vi "PH_IEEE1394Camera.set Cam Attributes to GUI.vi"(0 "VI in":refnum<vi>, 5 "error in (no error)":errorcluster) -> (14 "VI out":refnum<vi>, 19 "error out":errorcluster)   [LabVIEW 2014, in "PH_IEEE1394Camera.lvlib"]
uses:
  PH_IEEE1394Camera.lvlib
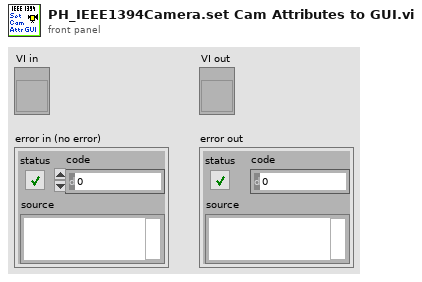
[diagram p1: front panel]
types:
  T1 = typedef "PH_IEEE1394Camera.lvlib/PH_IEEE1394Camera.i attribute.ctl" = cluster{"Gui Refs":cluster{"Brightness":refnum<vi>, "Shutter":refnum<vi>, "Gain":refnum<vi>, "Center of Gravity":refnum<vi>, "Supported Video Modes":refnum<vi>, "Trigger Polarity":refnum<vi>, "Trigger Mode":refnum<vi>, "Trigger Timeout":refnum<vi>, "Bit Depth":refnum<vi>, "Video Mode":refnum<vi>, "Top":refnum<vi>, "Bottom":refnum<vi>, "Left":refnum<vi>, "Right":refnum<vi>, "Set ROI to Maximum":refnum<vi>, "Camera Details":refnum<vi>, "Current Cam Attributes":refnum<vi>, "Attribute to set":refnum<vi>, "Num Value":refnum<vi>, "String Value":refnum<vi>, "Bool Value":refnum<vi>, "Set Cam Attribute":refnum<vi>}, "Cam":cluster{"IMAQ1394 Session":T2, "Camera Details":T3}, "Current Attributes":T4[], "Supported Video Modes ":cluster{"Video Mode":u32, "Video Mode Name":string}[], "Wanted Attributes":cluster{"Name":string, "Num Value":dbl, "String Value":string, "Boolean Value":bool}[], "Cam Attributes":T6}
  T2 = typedef "IMAQdx.ctl" = refnum<k21>
  T3 = typedef "PH_IEEE1394Camera.lvlib/PH_IEEE1394Camera.Cam Details.ctl" = cluster{"Model":string, "Serial Number":dbl, "Cam name (Machinery)":string, "Bus Type":string}
  T4 = typedef "PH_IEEE1394Camera.lvlib/PH_IEEE1394Camera.Cam Attribute.ctl" = cluster{"Information":cluster{"Type":T5, "Readable":bool, "Writable":bool, "Name":string}, "Num Value":dbl, "String Value":string, "Maximum":dbl, "Minimum":dbl, "Units":string, "Description":string, "EnumStrings[]":string[], "EnumValues[]":u32[], "Boolean Value":bool}
  T5 = typedef "NI_Vision_Acquisition_Software.lvlib/IMAQdx Attribute Type.ctl" = enum32{"U32", "I64", "DBL", "String", "Enum", "Bool", "Command"}
  T6 = typedef "PH_IEEE1394Camera.lvlib/PH_IEEE1394Camera.Relevant Cam Attributes.ctl" = cluster{"Video Mode":cluster{"Name":string, "Index":i32}, "Brightness":cluster{"Name":string, "Index":i32}, "Gain":cluster{"Name":string, "Index":i32}, "Shutter":cluster{"Name":string, "Index":i32}, "Trigger Pol":cluster{"Name":string, "Index":i32}, "Trigger Mode":cluster{"Name":string, "Index":i32}, "Timeout":cluster{"Name":string, "Index":i32}, "Bit Depth":cluster{"Name":string, "Index":i32}, "Pixel Bits":cluster{"Name":string, "Index":i32}, "Pixel Bytes":cluster{"Name":string, "Index":i32}, "Left":cluster{"Name":string, "Index":i32}, "Right":cluster{"Name":string, "Index":i32}, "Top":cluster{"Name":string, "Index":i32}, "Bottom":cluster{"Name":string, "Index":i32}}
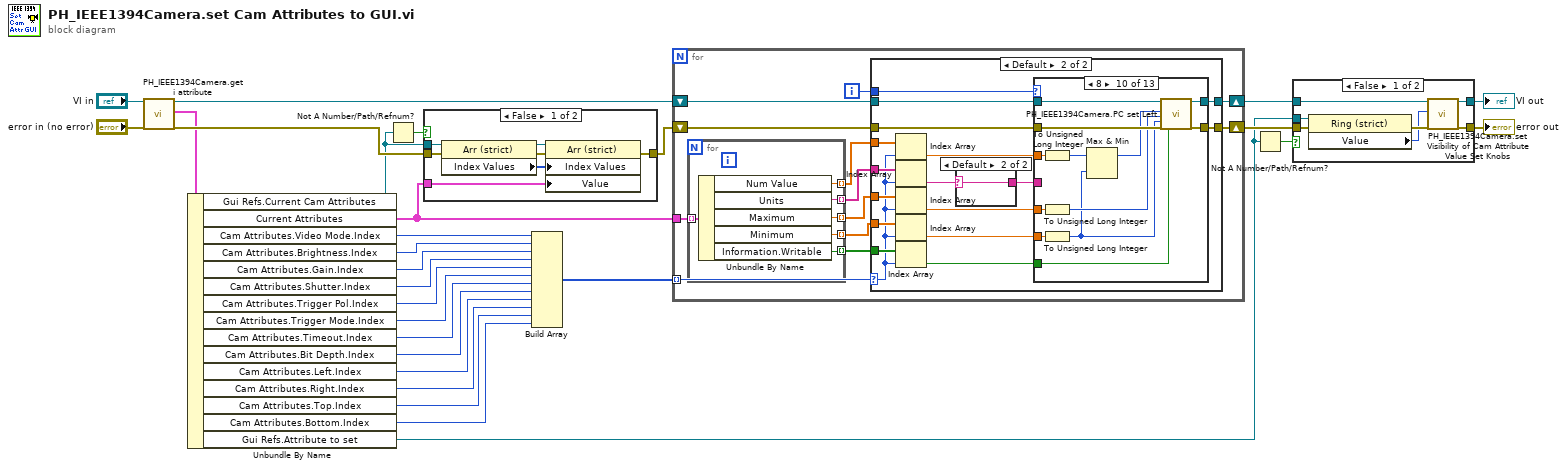
[diagram p0: block diagram]
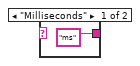
[diagram p4: hidden frame]
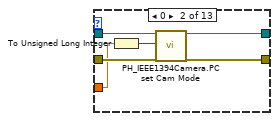
[diagram p6: hidden frame]
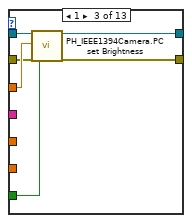
[diagram p7: hidden frame]
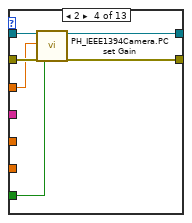
[diagram p8: hidden frame]
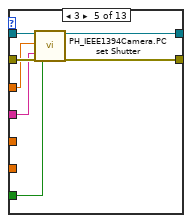
[diagram p9: hidden frame]
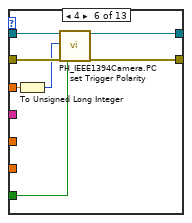
[diagram p10: hidden frame]
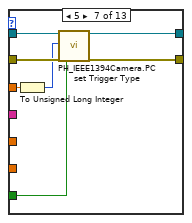
[diagram p11: hidden frame]
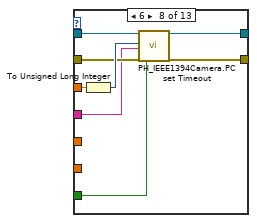
[diagram p12: hidden frame]
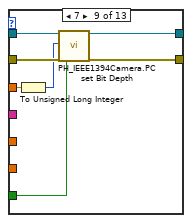
[diagram p13: hidden frame]
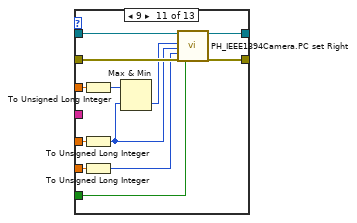
[diagram p14: hidden frame]
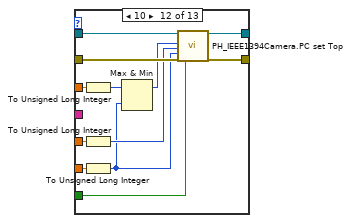
[diagram p15: hidden frame]
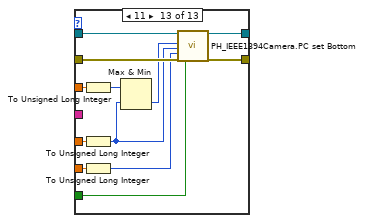
[diagram p16: hidden frame]
diagram:
  n1 = call "PH_IEEE1394Camera.get i attribute.vi"("i ref in"="VI in", "error in (no error)"="error in (no error)") -> ("i ref out"=w11:refnum<vi>, "i attribute"=w1:T1, "error out"=w14:errorcluster)  [unwired: 15 in]
  n2 = Unbundle By Name(w1) -> ("Gui Refs.Current Cam Attributes"=w13:refnum<vi>, "Current Attributes"=w9:T4[], "Cam Attributes.Video Mode.Index"=w26:i32, "Cam Attributes.Brightness.Index"=w25:i32, "Cam Attributes.Gain.Index"=w24:i32, "Cam Attributes.Shutter.Index"=w23:i32, "Cam Attributes.Trigger Pol.Index"=w22:i32, "Cam Attributes.Trigger Mode.Index"=w21:i32, "Cam Attributes.Timeout.Index"=w20:i32, "Cam Attributes.Bit Depth.Index"=w19:i32, "Cam Attributes.Left.Index"=w18:i32, "Cam Attributes.Right.Index"=w17:i32, "Cam Attributes.Top.Index"=w16:i32, "Cam Attributes.Bottom.Index"=w15:i32, "Gui Refs.Attribute to set"=w2:refnum<vi>)
  n3 = Not A Number/Path/Refnum?(number/path/refnum=w13) -> (NaN/Path/Refnum?=w12:bool)
  n4 = case shown="False" w12 {
    tunnel: [w32 w36] -> w10
    tunnel: w9 -> [w29 _]
    tunnel: w14 -> [w35 w36]
    tunnel: w13 -> [w34 _]
    frame False {
      n5 = property class="Arr (strict)"(reference=w34, error in=w35) -> (reference out=w30:refnum<vi>, error out=w33:errorcluster, "Index Values"=w31:u32[])
      n6 = property class="Arr (strict)"(reference=w30, error in=w33, "Index Values"=w31, "Value"=w29) -> (error out=w32:errorcluster)  [unwired: 1 out]
    }
    frame True {
    }
  }
  n7 = Build Array(w26, w25, w24, w23, w22, w21, w20, w19, w18, w17, w16, w15) -> (w8:i32[])
  n8 = for {
    shift-right: [w47] -> w7
    shift-left: w11 -> [w48]
    shift-right: [w46] -> w5
    shift-left: w10 -> [w45]
    tunnel: w9 -> [w44]
    tunnel: w8 -> [w38] mode=indexing
    i -> [w42]
    n9 = for {
      tunnel: w44 -> [w179] mode=indexing
      tunnel: [w178] -> w43 mode=indexing
      tunnel: [w177] -> w41 mode=indexing
      tunnel: [w176] -> w40 mode=indexing
      tunnel: [w175] -> w39 mode=indexing
      tunnel: [w174] -> w37 mode=indexing
      n10 = Unbundle By Name(w179) -> ("Num Value"=w178:dbl, "Units"=w174:string, "Maximum"=w176:dbl, "Minimum"=w175:dbl, "Information.Writable"=w177:bool)
    }
    n11 = case shown="Default" w38 {
      selector: w38 -> [_ w53]
      tunnel: w48 -> [w50 w67]
      tunnel: [w50 w66] -> w47
      tunnel: [w49 w65] -> w46
      tunnel: w45 -> [w49 w64]
      tunnel: w43 -> [_ w63]
      tunnel: w42 -> [_ w61]
      tunnel: w41 -> [_ w60]
      tunnel: w40 -> [_ w59]
      tunnel: w39 -> [_ w58]
      tunnel: w37 -> [_ w54]
      frame -1 {
      }
      frame Default {
        n12 = Index Array(array=w63, index=w53) -> (element=w62:dbl)
        n13 = Index Array(array=w54, index=w53) -> (element=w52:string)
        n14 = Index Array(array=w59, index=w53) -> (element=w57:dbl)
        n15 = Index Array(array=w58, index=w53) -> (element=w56:dbl)
        n16 = Index Array(array=w60, index=w53) -> (element=w55:bool)
        n17 = case shown="Default" w52 {
          selector: w52 -> [_ w69]
          tunnel: ["ms" w69] -> w51
          frame "Milliseconds" {
          }
          frame Default {
          }
        }
        n18 = case shown="8" w61 {
          tunnel: w67 -> [w71 w77 w81 w89 w96 w103 w110 w118 w125 w137 w149 w161 w173]
          tunnel: [w71 w76 w80 w87 w95 w102 w108 w114 w123 w135 w147 w159 w171] -> w66
          tunnel: [w70 w75 w79 w86 w93 w100 w107 w113 w122 w134 w146 w158 w170] -> w65
          tunnel: w64 -> [w70 w74 w82 w88 w94 w101 w109 w115 w124 w136 w148 w160 w172]
          tunnel: w62 -> [_ w73 w83 w85 w92 w99 w106 w117 w121 w133 w145 w157 w169]
          tunnel: w57 -> [_ _ _ _ _ _ _ _ _ w132 w144 w156 w168]
          tunnel: w56 -> [_ _ _ _ _ _ _ _ _ w131 w143 w155 w167]
          tunnel: w55 -> [_ _ w78 w84 w91 w97 w104 w112 w119 w129 w141 w153 w165]
          tunnel: w51 -> [_ _ _ _ w90 _ _ w111 _ _ _ _ _]
          frame Default {
          }
          frame 0 {
            n19 = To Unsigned Long Integer(number=w73) -> (unsigned 32bit integer=w72:u32)
            n20 = call "PH_IEEE1394Camera.PC set Cam Mode.vi"("i ref in"=w77, "Video Mode"=w72, "error in (no error)"=w74) -> ("i ref out"=w76:refnum<vi>, "error out"=w75:errorcluster)  [unwired: 15 in]
          }
          frame 1 {
            n21 = call "PH_IEEE1394Camera.PC set Brightness.vi"("i ref in"=w81, "Brightness"=w83, "error in (no error)"=w82, "Brightness writable? (True)"=w78) -> ("i ref out"=w80:refnum<vi>, "error out"=w79:errorcluster)  [unwired: 14 in]
          }
          frame 2 {
            n22 = call "PH_IEEE1394Camera.PC set Gain.vi"("i ref in"=w89, "Gain"=w85, "error in (no error)"=w88, "Gain writable? (True)"=w84) -> ("i ref out"=w87:refnum<vi>, "error out"=w86:errorcluster)  [unwired: 14 in]
          }
          frame 3 {
            n23 = call "PH_IEEE1394Camera.PC set Shutter.vi"("i ref in"=w96, "Shutter"=w92, "Unit"=w90, "error in (no error)"=w94, "Shutter writable? (True)"=w91) -> ("i ref out"=w95:refnum<vi>, "error out"=w93:errorcluster)  [unwired: 13 in]
          }
          frame 4 {
            n24 = To Unsigned Long Integer(number=w99) -> (unsigned 32bit integer=w98:u32)
            n25 = call "PH_IEEE1394Camera.PC set Trigger Polarity.vi"("i ref in"=w103, "Trigger Polarity"=w98, "error in (no error)"=w101, "Trigger Polarity writable? (True)"=w97) -> ("i ref out"=w102:refnum<vi>, "error out"=w100:errorcluster)  [unwired: 14 in]
          }
          frame 5 {
            n26 = To Unsigned Long Integer(number=w106) -> (unsigned 32bit integer=w105:u32)
            n27 = call "PH_IEEE1394Camera.PC set Trigger Type.vi"("i ref in"=w110, "Trigger Mode"=w105, "error in (no error)"=w109, "Trigger Mode writable? (True)"=w104) -> ("i ref out"=w108:refnum<vi>, "error out"=w107:errorcluster)  [unwired: 14 in]
          }
          frame 6 {
            n28 = To Unsigned Long Integer(number=w117) -> (unsigned 32bit integer=w116:u32)
            n29 = call "PH_IEEE1394Camera.PC set Timeout.vi"("i ref in"=w118, "Timeout"=w116, "Tip Strip"=w111, "error in (no error)"=w115, "Timeout writable? (True)"=w112) -> ("i ref out"=w114:refnum<vi>, "error out"=w113:errorcluster)  [unwired: 13 in]
          }
          frame 7 {
            n30 = To Unsigned Long Integer(number=w121) -> (unsigned 32bit integer=w120:u32)
            n31 = call "PH_IEEE1394Camera.PC set Bit Depth.vi"("i ref in"=w125, "Bit Depth"=w120, "error in (no error)"=w124, "Bit Depth writable? (True)"=w119) -> ("i ref out"=w123:refnum<vi>, "error out"=w122:errorcluster)  [unwired: 14 in]
          }
          frame 8 {
            n32 = To Unsigned Long Integer(number=w133) -> (unsigned 32bit integer=w127:u32)
            n33 = To Unsigned Long Integer(number=w132) -> (unsigned 32bit integer=w130:u32)
            n34 = To Unsigned Long Integer(number=w131) -> (unsigned 32bit integer=w128:u32)
            n35 = Max & Min(x=w127, y=w128) -> (max(x,y)=w126:u32)  [unwired: 1 out]
            n36 = call "PH_IEEE1394Camera.PC set Left.vi"("i ref in"=w137, "Left"=w126, "Maximum Left"=w130, "Minimum Left"=w128, "error in (no error)"=w136, "Left writable? (True)"=w129) -> ("i ref out"=w135:refnum<vi>, "error out"=w134:errorcluster)  [unwired: 12 in]
          }
          frame 9 {
            n37 = To Unsigned Long Integer(number=w145) -> (unsigned 32bit integer=w140:u32)
            n38 = To Unsigned Long Integer(number=w144) -> (unsigned 32bit integer=w139:u32)
            n39 = To Unsigned Long Integer(number=w143) -> (unsigned 32bit integer=w142:u32)
            n40 = Max & Min(x=w140, y=w139) -> (min(x,y)=w138:u32)  [unwired: 1 out]
            n41 = call "PH_IEEE1394Camera.PC set Right.vi"("i ref in"=w149, "Right"=w138, "Maximum Right"=w139, "Minimum Right"=w142, "error in (no error)"=w148, "Right writable? (True)"=w141) -> ("i ref out"=w147:refnum<vi>, "error out"=w146:errorcluster)  [unwired: 12 in]
          }
          frame 10 {
            n42 = To Unsigned Long Integer(number=w157) -> (unsigned 32bit integer=w152:u32)
            n43 = To Unsigned Long Integer(number=w156) -> (unsigned 32bit integer=w154:u32)
            n44 = To Unsigned Long Integer(number=w155) -> (unsigned 32bit integer=w151:u32)
            n45 = Max & Min(x=w152, y=w151) -> (max(x,y)=w150:u32)  [unwired: 1 out]
            n46 = call "PH_IEEE1394Camera.PC set Top.vi"("i ref in"=w161, "Top"=w150, "Maximum Top"=w154, "Minimum Top"=w151, "error in (no error)"=w160, "Top writable? (True)"=w153) -> ("i ref out"=w159:refnum<vi>, "error out"=w158:errorcluster)  [unwired: 12 in]
          }
          frame 11 {
            n47 = To Unsigned Long Integer(number=w169) -> (unsigned 32bit integer=w164:u32)
            n48 = To Unsigned Long Integer(number=w168) -> (unsigned 32bit integer=w163:u32)
            n49 = To Unsigned Long Integer(number=w167) -> (unsigned 32bit integer=w166:u32)
            n50 = Max & Min(x=w164, y=w163) -> (min(x,y)=w162:u32)  [unwired: 1 out]
            n51 = call "PH_IEEE1394Camera.PC set Bottom.vi"("i ref in"=w173, "Bottom"=w162, "Maximum Bottom"=w163, "Minimum Bottom"=w166, "error in (no error)"=w172, "Bottom writable? (True)"=w165) -> ("i ref out"=w171:refnum<vi>, "error out"=w170:errorcluster)  [unwired: 12 in]
          }
        }
      }
    }
  }
  n52 = Not A Number/Path/Refnum?(number/path/refnum=w2) -> (NaN/Path/Refnum?=w3:bool)
  n53 = case shown="False" w3 {
    tunnel: w7 -> [w186 w188]
    tunnel: [w185 w188] -> w6
    tunnel: w5 -> [w184 w187]
    tunnel: [w183 w187] -> w4
    tunnel: w2 -> [w181 _]
    frame False {
      n54 = property class="Ring (strict)"(reference=w181, error in=w184) -> (error out=w182:errorcluster, "Value"=w180:u32)  [unwired: 1 out]
      n55 = call "PH_IEEE1394Camera.set Visibility of Cam Attribute Value Set Knobs.vi"("VI in"=w186, "Index of selected Attribute"=w180, "error in (no error)"=w182) -> ("VI out"=w185:refnum<vi>, "error out"=w183:errorcluster)  [unwired: 15 in]
    }
    frame True {
    }
  }
  "error out" <- w4
  "VI out" <- w6
